vi "Set OutputPLC for Index.vi"(0 "Index":i32, 2 "Sat Coils":bool[](array[boolean])=[TRUE], 3 "error in (no error)":errorcluster) -> (10 "Error Out":errorcluster[](array[cluster]))   [LabVIEW 2019]
uses:
  Ctrl/Output to PLC.ctl
  Ctrl/S2 Station IO.ctl
  Ctrl/ModbusCmd.ctl
panel:
  in  "Array 3":T1=[enum."電流量測完成產品OK_21", enum."S2站Format 執行_23", enum."S2 Format OK_24"]
  in  "Array 2":T1=[enum."電流量測完成產品OK_21", enum."S2站Format 執行_23", enum."S2 Format OK_24"]
  in  "Address In":i32=20
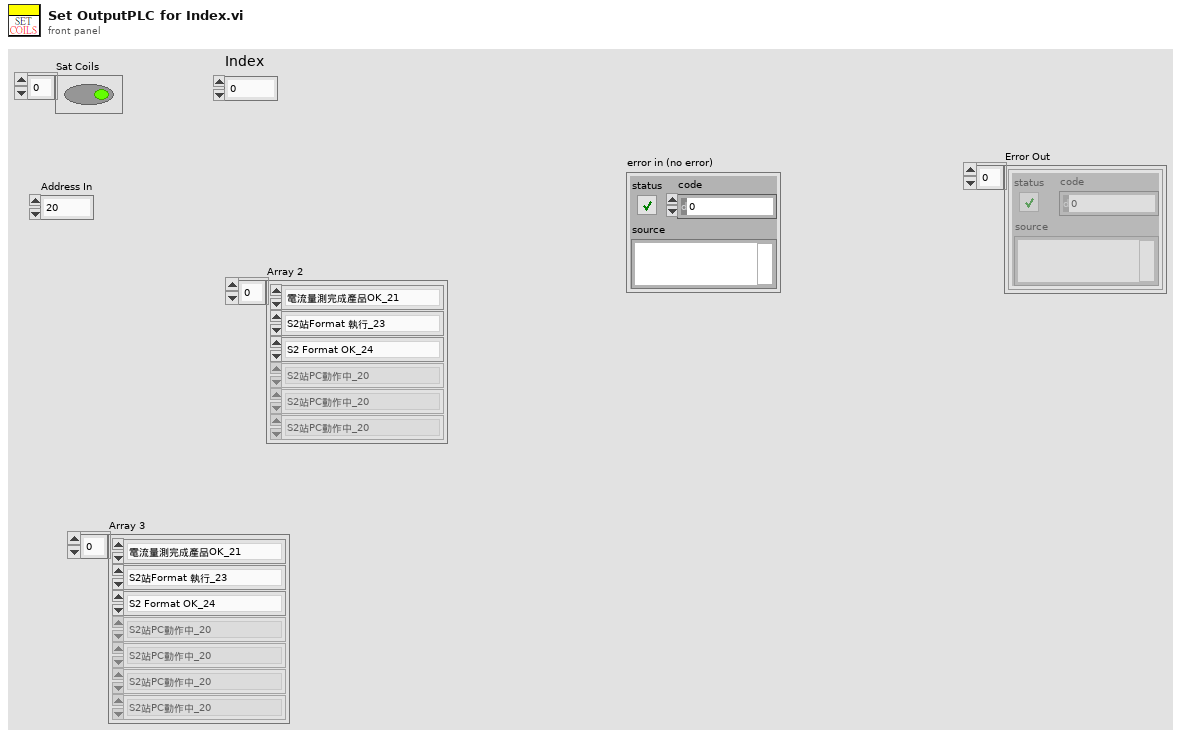
[diagram p1: front panel]
types:
  T1 = typedef "Output to PLC.ctl" = T2[]
  T2 = typedef "S2 Station IO.ctl" = enum16{"S2站PC動作中_20", "電流量測完成產品OK_21", "電流量測完成產品NG_22", "S2站Format 執行_23", "S2 Format OK_24", "S2 Format NG_25", "S2站燒入執行_26", "S2站燒入OK_27", "S2站燒入NG_28", "S2站動作完成_29", "S3 PC動作中_30", "S3 Format 此站執行_31", "S3 Format OK_32", "S3 Format NG_33", "S3 燒入程式 此站執行_34", "S3 燒入程式 OK_35", "S3 燒入程式 NG_36", "S3 備用_37", "S3 備用_38", "S3 動作完成_39", "S4 PC動作中_40", "S4 量測完成 產品正常_41", "S4 量測完成 產品NG_42", "S4 Format 此站執行_43", "S4 Format OK_44", "S4 Format NG_45", "S4 燒入 此站不執行_46", "S4 燒入程式 OK_47", "S4 燒入程式 NG_48", "S4 藍芽Scan OK_49", "S4 藍芽Scan NG_50", "S4 動作完成_51", "給PLC要量電流訊號", "給PLC要量電壓訊號"}
  T3 = cluster{"starting address":u16, "number of inputs":u16, "Sat Coils":bool[], "Holding Registers":u16[]}
  T4 = typedef "ModbusCmd.ctl" = enum16{"Connect", "Disconnect", "Init", "Fetch Basic Objects", "Fetch Input Refisters", "Fetch Discrete Inputs", "Set Coils", "Set Holding Registers", "Write Single Holding", "Exit"}
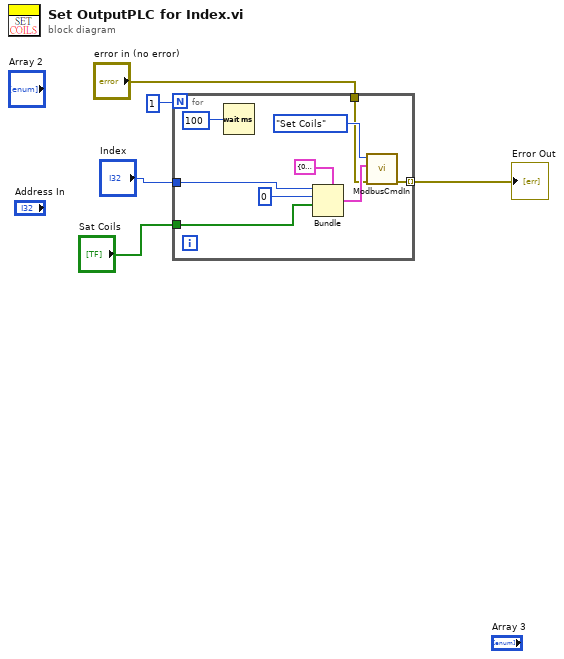
[diagram p0: block diagram]
diagram:
  n1 = for {
    N: 1 -> [_]
    tunnel: [w9] -> w5 mode=indexing
    tunnel: "Index" -> [w8]
    tunnel: "Sat Coils" -> [w7]
    tunnel: "error in (no error)" -> [w6]
    n2 = Wait (ms)(milliseconds to wait=100) -> ()  [unwired: 1 out]
    n3 = Bundle(cluster=T3 {"starting address"=0, "number of inputs"=0, "Sat Coils"=[], "Holding Registers"=[]} ("data"), "starting address"=w8, "number of inputs"=u16 0, "Sat Coils"=w7) -> (w12:T3)  [unwired: 1 in]
    n4 = call "ModbusCmdIn.vi"("error in (no error)"=w6, "data"=w12, "Enum"=ModbusCmd."Set Coils") -> ("error out"=w9:errorcluster)  [unwired: 8 in]
  }
  "Error Out" <- w5
